vi "Ellipiticity.vi"(2 "S":dbl, 3 "P":dbl) -> (0 "P+S":dbl, 1 "(P-S)/(P+S)":dbl)   [LabVIEW 2017, in "SignalConverson.lvlib"]
uses:
  SignalConverson.lvlib
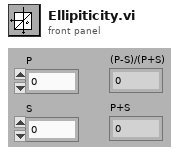
[diagram p1: front panel]
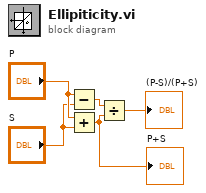
[diagram p0: block diagram]
diagram:
  n1 = Subtract(x="P", y="S") -> (x-y=w2:dbl)
  n2 = Add(x="P", y="S") -> (x+y=w1:dbl)
  "P+S" <- w1
  n3 = Divide(x=w2, y=w1) -> (x/y=→"(P-S)/(P+S)":dbl)
